vi "Pre-Build VI - Run Unit Tests.vi"(8 "error in (no error)":errorcluster) -> (0 "error out":errorcluster, 1 "VIs without test coverage":string[](array[string]), 2 "error type":enum16{"fatal", "non-fatal", "warning"}(ring), 3 "num_tests":i32, 4 "VIs not loadable":string[](array[string]))   [LabVIEW 2020]
panel:
  out "VIs Failed":string[](array[string])
  out "VIs Succeeded":string[](array[string])
  in  "type specifier VI Refnum (for type only)":refnum<vi>
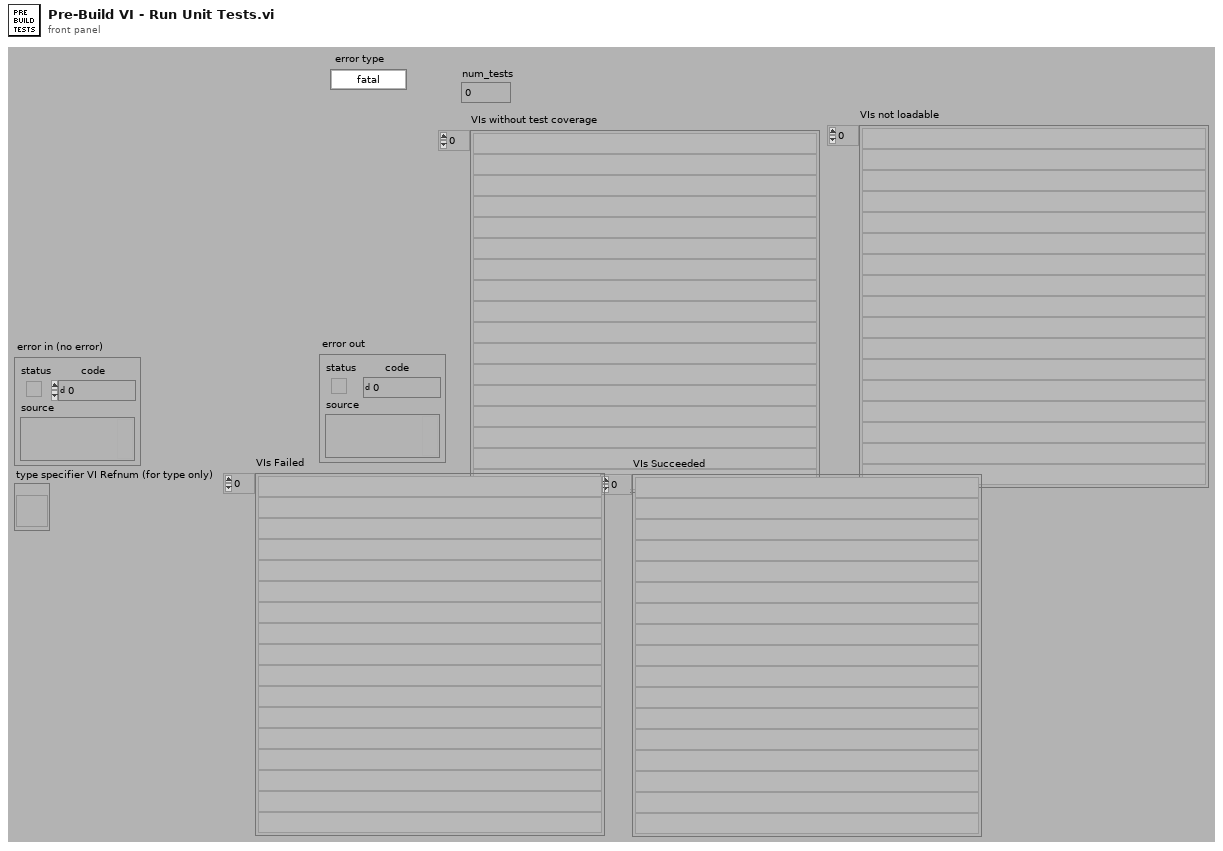
[diagram p1: front panel]
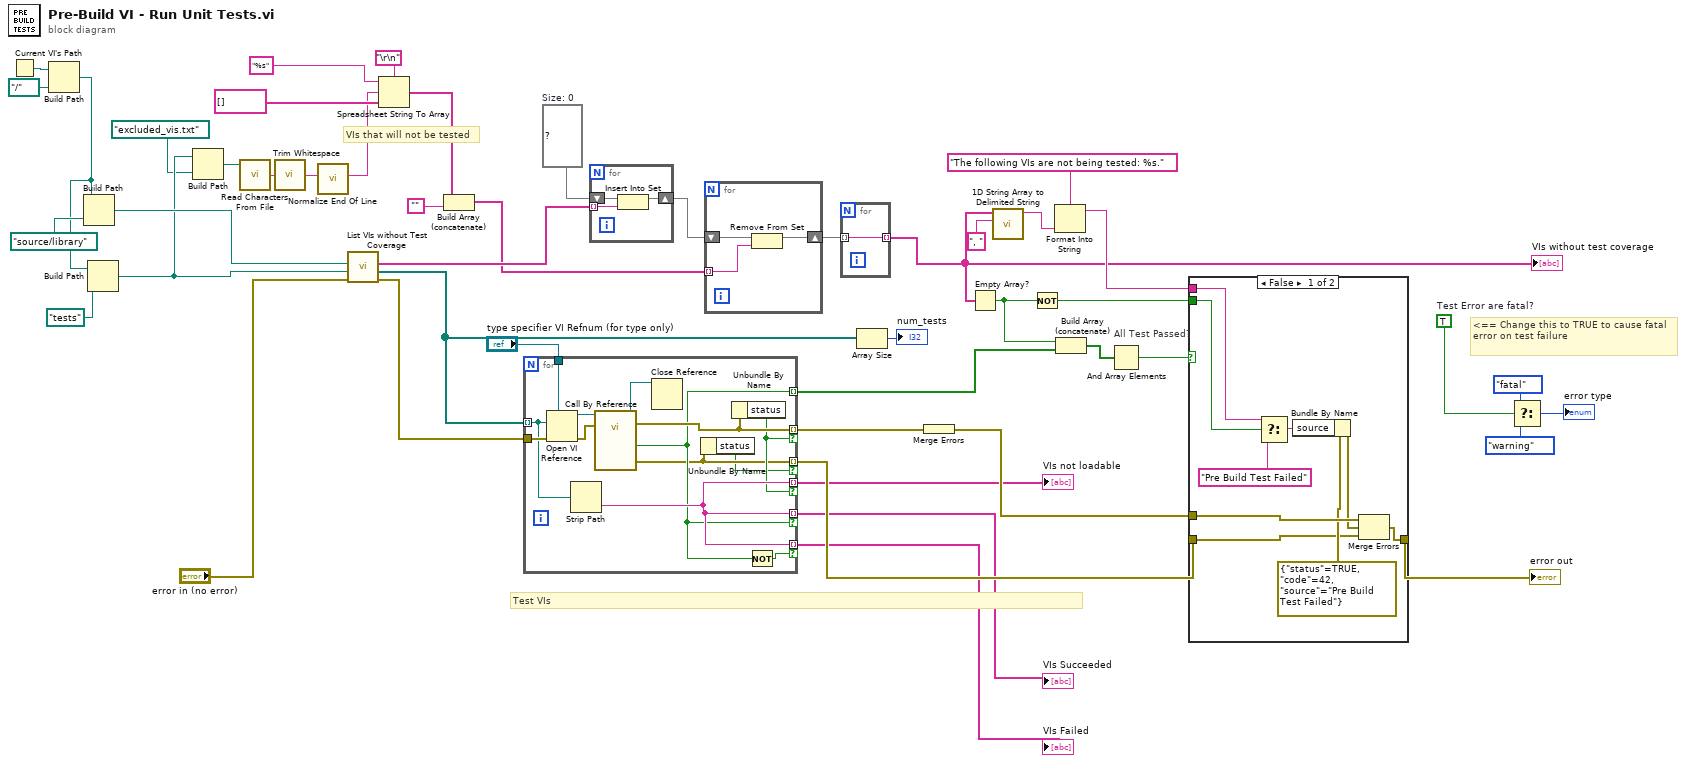
[diagram p0: block diagram]
diagram:
  w15 = set{string} {}  # Size: 0
  w38 = TRUE  # Test Error are fatal?
  # "VIs that will not be tested"
  # "<== Change this to TRUE to cause fatal error on test failure"
  # "All Test Passed?"
  # "Test VIs"
  n1 = Current VI's Path() -> (path=w24:path)
  n2 = Build Path(base path=w24, name or relative path=path "../..") -> (appended path=w20:path)
  n3 = Build Path(base path=w20, name or relative path=path "source/library" ("Relative path (.)")) -> (appended path=w22:path)
  n4 = Build Path(base path=w20, name or relative path=path "tests" ("Relative path (.)")) -> (appended path=w18:path)
  n5 = Build Path(base path=w18, name or relative path=path "excluded_vis.txt" ("Relative path (.)")) -> (appended path=w16:path)
  n6 = call <vilib>:"Read Characters From File.vi"("file path (dialog if empty)"=w16) -> ("character string"=w6:string)  [unwired: 5 in, 3 out]
  n7 = call <vilib>:"Trim Whitespace.vi"("string"=w6) -> ("trimmed string"=w4:string)  [unwired: 1 in]
  n8 = call <vilib>:"Normalize End Of Line.vi"("string in"=w4) -> ("string out"=w3:string)  [unwired: 7 in]
  n9 = call "List VIs without Test Coverage.vi"("error in (no error)"="error in (no error)", "Tests Root"=w18, "Source Root"=w22) -> ("error out"=w31:errorcluster, "Test VIs"=w2:path[], "VIs without test coverage"=w14:string[])  [unwired: 6 in]
  n10 = Spreadsheet String To Array(delimiter (Tab)="\r\n", format string="%s", spreadsheet string=w3, array type (2D Dbl)=string[] [] ("appended array")) -> (array=w5:string[])
  n11 = Build Array (concatenate)(w5, "") -> (w12:string[])
  n12 = for {
    tunnel: w2 -> [w55] mode=indexing
    tunnel: "type specifier VI Refnum (for type only)" -> [w61]
    tunnel: [w53] -> w28 mode=indexing
    tunnel: [w50] -> w33 mode=indexing if=w49
    tunnel: w31 -> [w57]
    tunnel: [w56] -> w29 mode=indexing if=w51
    tunnel: [w54] -> w27 mode=indexing if=w51
    tunnel: [w54] -> w26 mode=indexing if=w53
    tunnel: [w54] -> w25 mode=indexing if=w52
    n13 = Open VI Reference(type specifier VI Refnum (for type only)=w61, vi path=w55, error in (no error)=w57) -> (vi reference=w60:refnum<vi>, error out=w59:errorcluster)  [unwired: 3 in]
    n14 = Strip Path(path=w55) -> (name=w54:string)  [unwired: 1 out]
    n15 = call-by-ref "?"(reference=w60, error in=w59) -> (reference out=w58:refnum<vi>, error out=w56:errorcluster, 0:"error out"=w50:errorcluster, "pass"=w53:bool)  [unwired: 10 in]
    n16 = Close Reference(reference=w58) -> ()  [unwired: 1 in, 1 out]
    n17 = Unbundle By Name(w50) -> ("status"=w49:bool)
    n18 = Unbundle By Name(w56) -> ("status"=w51:bool)
    n19 = Not(x=w53) -> (.not. x?=w52:bool)
  }
  "VIs not loadable" <- w27
  "VIs Succeeded" <- w26
  "VIs Failed" <- w25
  n20 = for {
    tunnel: w14 -> [w64] mode=indexing
    shift-right: [w62] -> w13
    shift-left: w15 -> [w63]
    n21 = Insert Into Set(10:w64, 11:w63) -> (3:w62:set{string})  [unwired: 1 out]
  }
  n22 = for {
    shift-right: [w65] -> w11
    shift-left: w13 -> [w67]
    tunnel: w12 -> [w66] mode=indexing
    n23 = Remove From Set(10:w66, 11:w67) -> (3:w65:set{string})  [unwired: 1 out]
  }
  n24 = for {
    tunnel: [w68] -> w10 mode=indexing
    tunnel: w11 -> [w68] mode=indexing
  }
  "VIs without test coverage" <- w10
  n25 = Array Size(array=w2) -> (size(s)=→"num_tests":i32)
  n26 = Merge Errors(w29) -> (w30:errorcluster)
  n27 = Empty Array?(array=w10) -> (empty?=w42:bool)
  n28 = call <vilib>:"1D String Array to Delimited String.vi"("delimiter"=", " ("delimiter (Tab)"), "string array"=w10) -> ("delimited string"=w45:string)  [unwired: 9 in]
  n29 = Not(x=w42) -> (.not. x?=w41:bool)
  n30 = Format Into String(format string="The following VIs are not being tested: %s.", w45) -> (resulting string=w43:string)  [unwired: 2 in, 1 out]
  n31 = Build Array (concatenate)(w42, w28) -> (w48:bool[])
  n32 = And Array Elements(Boolean array=w48) -> (logical AND=w47:bool)
  n33 = case shown="False" w47 {
    tunnel: w30 -> [w77 w78]
    tunnel: [w76 w78] -> w40
    tunnel: w41 -> [w75 _]
    tunnel: w43 -> [w74 _]
    tunnel: w33 -> [w69 _]
    frame False {
      n34 = Select(t=w74, s=w75, f="Pre Build Test Failed" ("source")) -> (s? t:f=w72:string)
      n35 = Bundle By Name(cluster=errorcluster {"status"=TRUE, "code"=42, "source"="Pre Build Test Failed"} ("error out"), "source"=w72) -> (w71:errorcluster)
      n36 = Merge Errors(w77, w71, w69) -> (w76:errorcluster)
    }
    frame True {
    }
  }
  "error out" <- w40
  n37 = Select(t=enum16{"fatal", "non-fatal", "warning"}."fatal" ("error type"), s=w38, f=enum16{"fatal", "non-fatal", "warning"}."warning" ("error type")) -> (s? t:f=→"error type":enum16{"fatal", "non-fatal", "warning"})
